vi "Actor Core.vi"(8 "error in":errorcluster, 11 "Smart Relay in":refnum<class "Smart Relay.lvclass">) -> (0 "error out":errorcluster, 3 "Actor out":refnum<class "Actor.lvclass">)   [LabVIEW 2018, in "Smart Relay Actor.lvlib" / "Smart Relay.lvclass"]
doc: "(<B>Filename</B>: Actor Framework.lvlib:Actor.lvclass:Actor Core.vi)\n\nReceives messages to the actor, reacts to them, and initiates any error handling that may shut the actor down.\n\nDescendant classes may override this VI to append parallel tasks for the actor to complete while it handles messages. Overrides use the Call Parent Method node."
uses:
  Smart Relay.lvclass
  C:/Users/Administrator/Desktop/2018LabVIEW EMS/EMS Generic Actor/EMS Generic/EMS Generic.lvclass
  <vilib>/ActorFramework/Actor/Actor.lvclass
  EMS Generic Actor/EMS Generic/EMS Generic.lvclass/EMS Generic.ctl
  <vilib>/ORNL/CSEISMIC DDS/CSEISMIC DDS Base/CSEISMIC DDS.lvclass/CSEISMIC DDS.ctl
  <vilib>/ORNL/CSEISMIC DDS/CSEISMIC DDS Base/Accessors/Write DDS Reference.vi
  <vilib>/ORNL/CSEISMIC DDS/CSEISMIC DDS Base/Accessors/Read DDS Reference.vi
  <vilib>/ORNL/CSEISMIC DDS/DDS Reader/DDS Reader.lvclass
  C:/Program Files (x86)/National Instruments/LabVIEW 2018/vi.lib/ORNL/CSEISMIC DDS/CSEISMIC DDS Base/CSEISMIC DDS.lvclass
  <vilib>/ORNL/CSEISMIC DDS/CSEISMIC DDS Base/Error Handler.vi
  Device DDS Communications Framework/Device DDS Communications/Device DDS Communications.lvclass
  EMS Generic Actor/EMS Generic/EMS Generic.lvclass
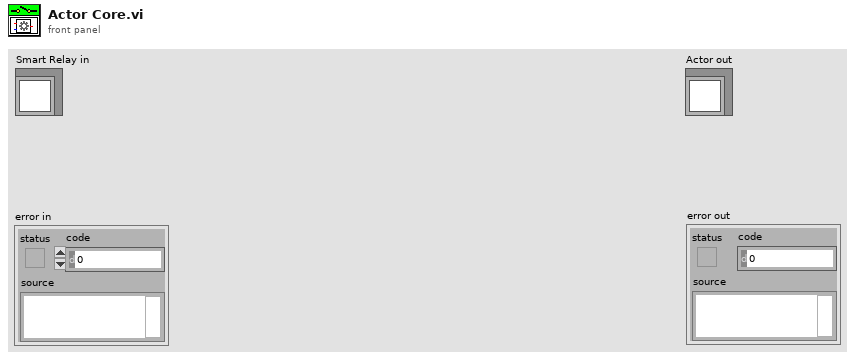
[diagram p1: front panel]
types:
  T1 = typedef "CSEISMIC DDS.lvlib/CSEISMIC DDS.lvclass/DeviceID.ctl" = string
  T2 = typedef "CSEISMIC DDS.lvlib/CSEISMIC DDS.lvclass/SmartRelay_Measurement.ctl" = cluster{"DeviceID":T1, "PrimaryVoltage":dbl[], "SecondaryVoltage":dbl[], "Current":dbl[], "RealPower":dbl[], "ReactivePower":dbl[], "LineConfig":u8[], "Frequency":dbl}
  T3 = typedef "LVDDS_library.lvlib/DDS Sample Info.ctl" = cluster{"DDS_SampleStateKind":enum32{"DDS_INVALID_SAMPLE_STATE", "DDS_READ_SAMPLE_STATE", "DDS_NOT_READ_SAMPLE_STATE"}, "DDS_ViewStateKind":enum32{"DDS_INVALID_SAMPLE_STATE", "DDS_NEW_VIEW_STATE", "DDS_NOT_NEW_VIEW_STATE"}, "DDS_InstanceStateKind":enum32{"DDS_INVALID_STATE", "DDS_ALIVE_INSTANCE_STATE", "DDS_NOT_ALIVE_DISPOSED_INSTANCE_STATE", "", "DDS_NOT_ALIVE_NO_WRITERS_INSTANCE_STATE"}, "sec":i32, "nanosec":u32, "valid_data":bool}
  T4 = typedef "CSEISMIC DDS.lvlib/CSEISMIC DDS.lvclass/SmartRelay_Info.ctl" = cluster{"DeviceID":T1, "LineConfig":u8[], "NominalVoltage(V)":dbl}
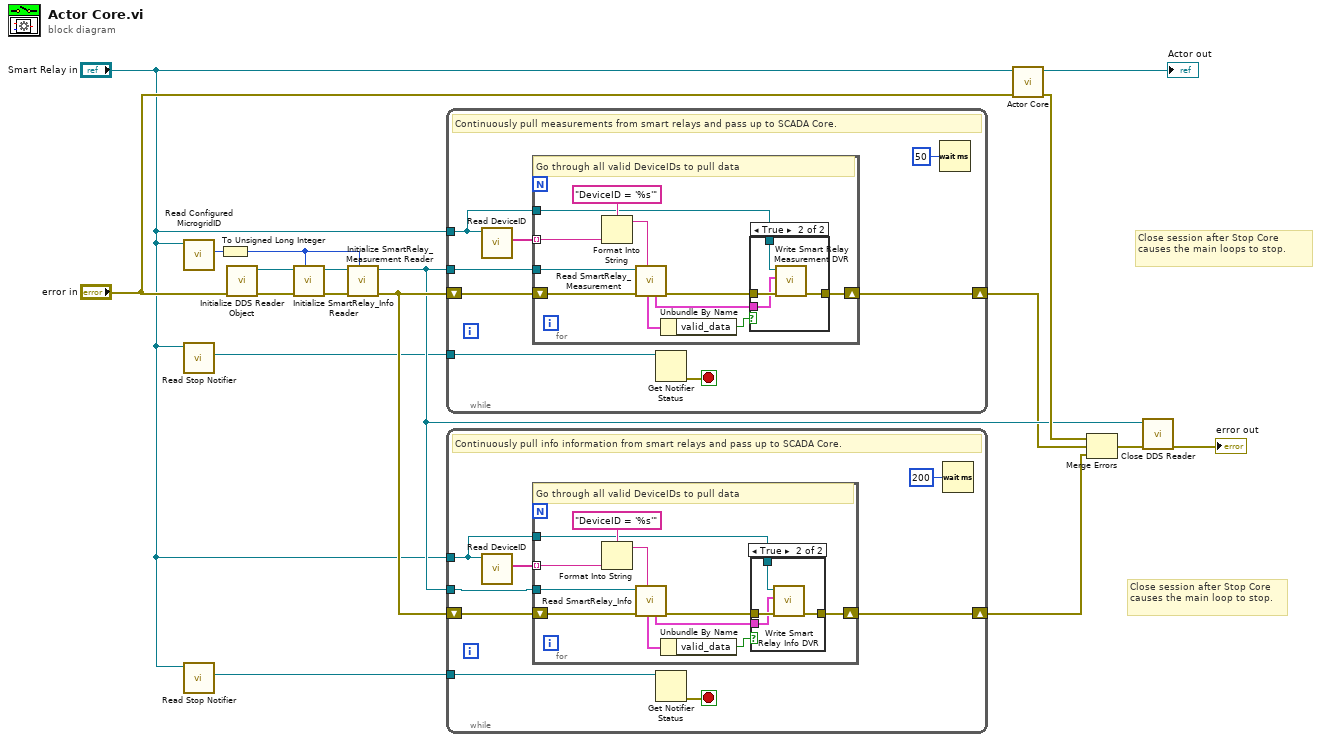
[diagram p0: block diagram]
diagram:
  # "Close session after Stop Core causes the main loop to stop."
  # "Close session after Stop Core causes the main loops to stop."
  n1 = call "Read Configured MicrogridID.vi"("EMS Generic in"="Smart Relay in") -> ("Microgrid ID"=w18:u8)  [unwired: 8 in, 2 out]
  n2 = call "Read Stop Notifier.vi"("EMS Generic in"="Smart Relay in") -> ("stop"=w6:refnum<notifier>)  [unwired: 9 in, 1 out]
  n3 = call "Read Stop Notifier.vi"("EMS Generic in"="Smart Relay in") -> ("stop"=w7:refnum<notifier>)  [unwired: 9 in, 1 out]
  n4 = To Unsigned Long Integer(number=w18) -> (unsigned 32bit integer=w8:u32)
  n5 = call <vilib>:"Initialize DDS Reader Object.vi"("error in"="error in") -> ("error out"=w14:errorcluster, "DDS Reader out"=w13:refnum<class "DDS Reader.lvclass">)  [unwired: 9 in]
  n6 = call <vilib>:"Initialize SmartRelay_Info Reader.vi"("MicrogridID"=w8, "error in"=w14, "DDS Reader in"=w13) -> ("error out"=w15:errorcluster, "DDS Reader out"=w12:refnum<class "DDS Reader.lvclass">)  [unwired: 7 in]
  n7 = call <vilib>:"Initialize SmartRelay_Measurement Reader.vi"("MicrogridID"=w8, "error in"=w15, "DDS Reader in"=w12) -> ("error out"=w11:errorcluster, "DDS Reader out"=w10:refnum<class "DDS Reader.lvclass">)  [unwired: 7 in]
  n8 = while {
    tunnel: w6 -> [w26]
    shift-right: [w20] -> w3
    shift-left: w11 -> [w22]
    tunnel: "Smart Relay in" -> [w19]
    tunnel: w10 -> [w21]
    stop <- w25 stop-if-true
    # "Continuously pull measurements from smart relays and pass up to SCADA Core."
    n9 = call-dynamic "Read DeviceID.vi"("Device DDS Communications in"=w19) -> ("DeviceID"=w23:T1[])  [unwired: 9 in, 1 out]
    n10 = for {
      shift-right: [w28] -> w20
      shift-left: w22 -> [w36]
      tunnel: w23 -> [w34] mode=indexing
      tunnel: w21 -> [w37]
      tunnel: w19 -> [w27]
      # "Go through all valid DeviceIDs to pull data"
      n11 = Format Into String(format string="DeviceID = '%s'", w34) -> (resulting string=w33:string)  [unwired: 2 in, 1 out]
      n12 = call <vilib>:"Read SmartRelay_Measurement.vi"("Query condition"=w33, "error in"=w36, "DDS Reader in"=w37) -> ("error out"=w29:errorcluster, "data"=w30:T2, "DDS Sample Info"=w32:T3)  [unwired: 5 in, 1 out]
      n13 = Unbundle By Name(w32) -> ("valid_data"=w31:bool)
      n14 = case shown="True" w31 {
        tunnel: w30 -> [_ w39]
        tunnel: w29 -> [w38 w42]
        tunnel: [w38 w41] -> w28
        tunnel: w27 -> [_ w40]
        frame False {
        }
        frame True {
          n15 = call "Write Smart Relay Measurement DVR.vi"("error in"=w42, "SmartRelay_Measurement"=w39, "EMS Generic in"=w40) -> ("error out"=w41:errorcluster)  [unwired: 7 in, 1 out]
        }
      }
    }
    n16 = Get Notifier Status(notifier=w26) -> (error out=w25:errorcluster)  [unwired: 1 in, 4 out]
    n17 = Wait (ms)(milliseconds to wait=u32 50) -> ()  [unwired: 1 out]
  }
  n18 = while {
    tunnel: w7 -> [w50]
    shift-right: [w44] -> w2
    shift-left: w11 -> [w46]
    tunnel: "Smart Relay in" -> [w43]
    tunnel: w10 -> [w45]
    stop <- w49 stop-if-true
    # "Continuously pull info information from smart relays and pass up to SCADA Core."
    n19 = call-dynamic "Read DeviceID.vi"("Device DDS Communications in"=w43) -> ("DeviceID"=w47:T1[])  [unwired: 9 in, 1 out]
    n20 = for {
      shift-right: [w52] -> w44
      shift-left: w46 -> [w60]
      tunnel: w47 -> [w58] mode=indexing
      tunnel: w45 -> [w61]
      tunnel: w43 -> [w51]
      # "Go through all valid DeviceIDs to pull data"
      n21 = Format Into String(format string="DeviceID = '%s'", w58) -> (resulting string=w57:string)  [unwired: 2 in, 1 out]
      n22 = call <vilib>:"Read SmartRelay_Info.vi"("Query condition"=w57, "error in"=w60, "DDS Reader in"=w61) -> ("error out"=w53:errorcluster, "data"=w54:T4, "DDS Sample Info"=w56:T3)  [unwired: 5 in, 1 out]
      n23 = Unbundle By Name(w56) -> ("valid_data"=w55:bool)
      n24 = case shown="True" w55 {
        tunnel: w54 -> [_ w63]
        tunnel: w53 -> [w62 w66]
        tunnel: [w62 w65] -> w52
        tunnel: w51 -> [_ w64]
        frame False {
        }
        frame True {
          n25 = call "Write Smart Relay Info DVR.vi"("error in"=w66, "SmartRelay_Info"=w63, "EMS Generic in"=w64) -> ("error out"=w65:errorcluster)  [unwired: 7 in, 1 out]
        }
      }
    }
    n26 = Get Notifier Status(notifier=w50) -> (error out=w49:errorcluster)  [unwired: 1 in, 4 out]
    n27 = Wait (ms)(milliseconds to wait=u32 200) -> ()  [unwired: 1 out]
  }
  n28 = call-parent "Actor Core.vi"("error in"="error in", "Actor in"="Smart Relay in") -> ("error out"=w17:errorcluster, "Actor out"=→"Actor out":refnum<class "Actor.lvclass">)  [unwired: 8 in]
  n29 = Merge Errors(w17, w3, w2) -> (w5:errorcluster)
  n30 = call <vilib>:"Close DDS Reader.vi"("error in"=w5, "DDS Reader in"=w10) -> ("error out"=→"error out":errorcluster)  [unwired: 9 in]
